vi "Create Main DataTransfer Queues.vi"(8 "error in (no error)":errorcluster, 11 "Main in":refnum<class "Main.lvclass">) -> (0 "error out":errorcluster, 1 "DPAuxDataQ":T1, 2 "InverterWaveformsQ-DT":T2, 3 "Main out":refnum<class "Main.lvclass">)   [LabVIEW 2019, in "Main.lvclass"]
doc: "Developed by Kevin Thompson\nkevin@thompsonengineering.net\n\nCopyright 2020\nThompson Engineering, LLC"
uses:
  Main.lvclass
  Common/DataTypes/ChannelWaveforms--cluster.ctl
  Common/DataTypes/InverterWaveforms--cluster.ctl
  Common/DataTypes/InverterWaveforms--QRef.ctl
  DataTypes/DataProcessAuxData--cluster.ctl
  Common/DataTypes/DataProcAuxDat--Qref.ctl
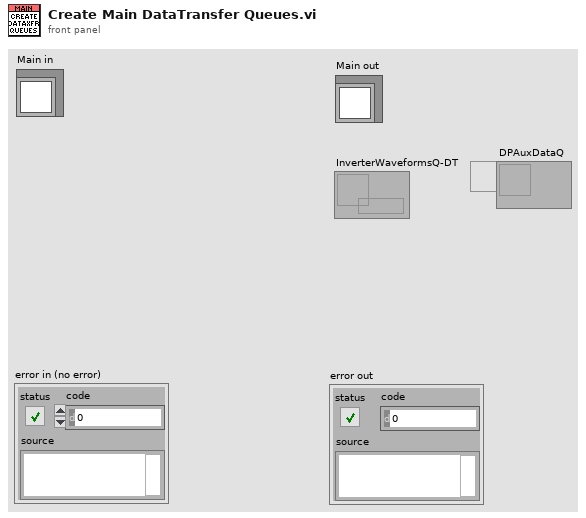
[diagram p1: front panel]
types:
  T1 = typedef "DataProcAuxDat--Qref.ctl" = refnum<queue>
  T2 = typedef "InverterWaveforms--QRef.ctl" = refnum<queue>
  T3 = typedef "DataProcessAuxData--cluster.ctl" = cluster{"Time Stamp":timestamp, "Raw ESR sum":dbl, "Inv 1 ON?":bool, "Average scaled ESR sum":dbl, "Inv 1 over threshold?":bool, "Inv 1 ESR":cluster{"ESR Baseline":dbl, "Alarm threshhold (%)":dbl, "Avg value":dbl}, "Max ESR":dbl}
  T4 = typedef "InverterWaveforms--cluster.ctl" = T5[]
  T5 = typedef "ChannelWaveforms--cluster.ctl" = cluster{"Iin ripple ":waveform(dbl), "Iout ripple ":waveform(dbl), "Iout 60Hz":waveform(dbl), "Vout 60Hz":waveform(dbl)}
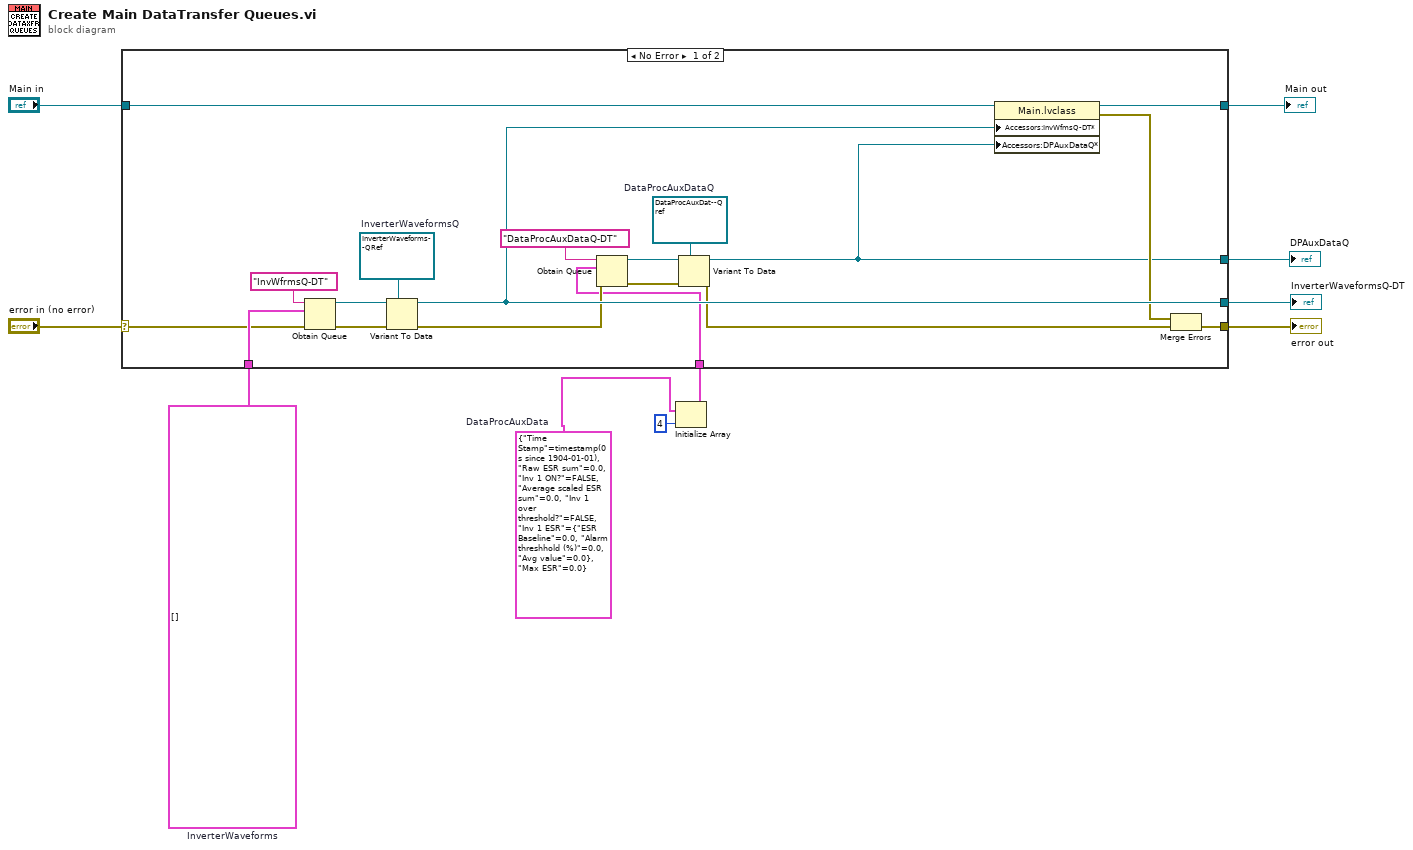
[diagram p0: block diagram]
diagram:
  w3 = T3 {"Time Stamp"=timestamp(0 s since 1904-01-01), "Raw ESR sum"=0.0, "Inv 1 ON?"=FALSE, "Average scaled ESR sum"=0.0, "Inv 1 over threshold?"=FALSE, "Inv 1 ESR"={"ESR Baseline"=0.0, "Alarm threshhold (%)"=0.0, "Avg value"=0.0}, "Max ESR"=0.0}  # DataProcAuxData
  w4 = T4 []  # InverterWaveforms
  n1 = Initialize Array(w3, 4 ("dimension size")) -> (w1:T3[])
  n2 = case shown="No Error" "error in (no error)" {
    selector: "error in (no error)" -> [w26 w31]
    tunnel: [w23 _] -> w10
    tunnel: w4 -> [w29 _]
    tunnel: [w22 w31] -> w9
    tunnel: "Main in" -> [w25 w30]
    tunnel: [w24 w30] -> w6
    tunnel: [w15 _] -> w5
    tunnel: w1 -> [w11 _]
    frame No Error {
      w17 = T1 refnum  # DataProcAuxDataQ
      w28 = T2 refnum  # InverterWaveformsQ
      n3 = Obtain Queue(name (unnamed)="InvWfrmsQ-DT", element data type=w29, error in (no error)=w26) -> (queue out=w12:refnum<queue>, error out=w27:errorcluster)  [unwired: 2 in, 1 out]
      n4 = Variant To Data(error in=w27, type=w28, Variant=w12) -> (data=w23:T2, error out=w13:errorcluster)
      n5 = Obtain Queue(name (unnamed)="DataProcAuxDataQ-DT", element data type=w11, error in (no error)=w13) -> (queue out=w16:refnum<queue>, error out=w19:errorcluster)  [unwired: 2 in, 1 out]
      n6 = Variant To Data(error in=w19, type=w17, Variant=w16) -> (data=w15:T1, error out=w14:errorcluster)
      n7 = property class="Main.lvclass"(reference=w25, "Accessors:InvWfmsQ-DT*"=w23, "Accessors:DPAuxDataQ*"=w15) -> (reference out=w24:refnum<class "Main.lvclass">, error out=w21:errorcluster)  [unwired: 1 in]
      n8 = Merge Errors(w21, w14) -> (w22:errorcluster)
    }
    frame Error {
    }
  }
  "InverterWaveformsQ-DT" <- w10
  "error out" <- w9
  "Main out" <- w6
  "DPAuxDataQ" <- w5
